vi "AcknowledgeInterrupts.vi"(8 "error in (no error)":errorcluster, 11 "BME_DG_Base in":refnum<class "BME_DG_Base.lvclass">) -> (0 "error out":errorcluster, 3 "BME_DG_Base out":refnum<class "BME_DG_Base.lvclass">)   [LabVIEW 2009, in "BME_DG_Base.lvclass"]
uses:
  BME_DG_Base.lvclass
  BME_DG_Base.lvclass/BME_DG_Base.ctl
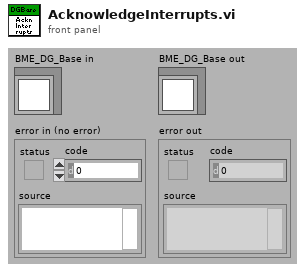
[diagram p1: front panel]
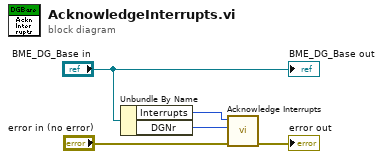
[diagram p0: block diagram]
diagram:
  n1 = Unbundle By Name("BME_DG_Base in") -> ("Interrupts"=w1:u32, "DGNr"=w2:i32)
  n2 = call "Acknowledge Interrupts.vi"("error in (no error)"="error in (no error)", "DG Number"=w2, "Interrupt Ack"=w1) -> ("error out"=→"error out":errorcluster)  [unwired: 8 in]
  "BME_DG_Base out" <- "BME_DG_Base in"
